vi "Fetch Single Measurement (Current Harmonics).vi"(0 "VISA resource name":refnum<visa-resource-name>, 7 "Harmonic Order (1)":u8=1, 9 "Phase Order (1)":u8=1, 11 "error in (no error)":errorcluster) -> (3 "Total Current Harmonic Distortion":dbl, 4 "VISA resource name out":refnum<visa-resource-name>, 6 "Current Crestfactor":dbl, 8 "Nth Current Harmonic Amplitude":dbl, 10 "Nth Current Harmonic Phase":dbl, 15 "error out":errorcluster)   [LabVIEW 2020, in "Agilent 681x Series.lvlib"]
doc: "Fetches and returns the selected order harmonic amplitude and phase measurements, the crestfactor of the waveform and the total harmonic distortion.\n\n<B>Note:</B>\n\nUse this VI only with other low-level VIs. The high-level VIs automatically incorporate this functionality. This VI does not check the instrument status. If you want to check the instrument status, call the Error Query VI at the conclusion of the sequence."
uses:
  <instrlib>/Agilent 681x Series/Agilent 681x Series.lvlib
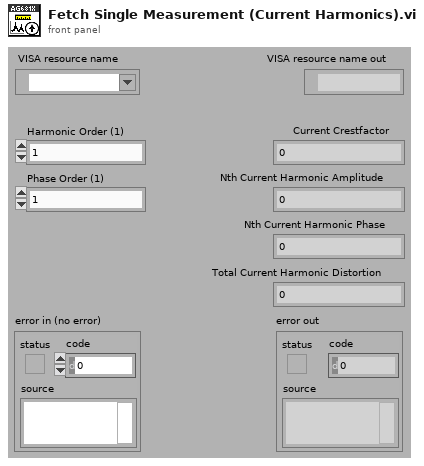
[diagram p1: front panel]
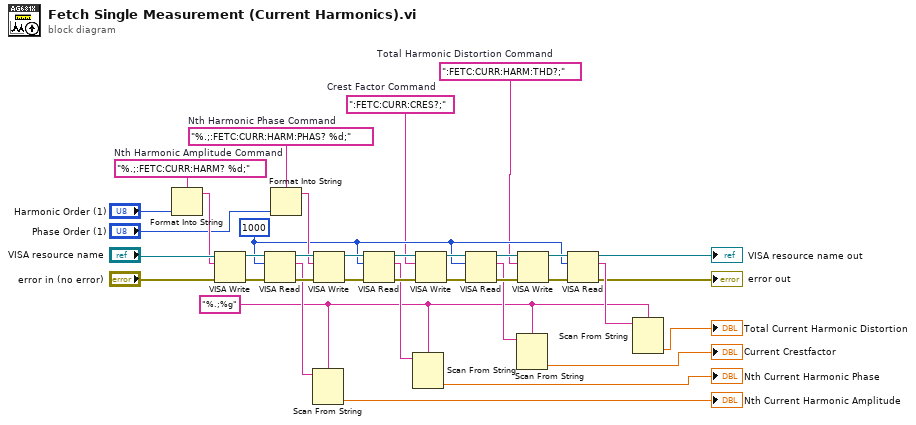
[diagram p0: block diagram]
diagram:
  w4 = "%.;%g" ("format string")
  w13 = ":FETC:CURR:CRES?;"  # Crest Factor Command
  w19 = "%.;:FETC:CURR:HARM:PHAS? %d;"  # Nth Harmonic Phase Command
  w20 = "%.;:FETC:CURR:HARM? %d;"  # Nth Harmonic Amplitude Command
  w14 = u32 1000 ("byte count")
  w12 = ":FETC:CURR:HARM:THD?;"  # Total Harmonic Distortion Command
  n1 = Format Into String(format string=w20, "Harmonic Order (1)") -> (resulting string=w17:string)  [unwired: 2 in, 1 out]
  n2 = VISA Write(VISA resource name="VISA resource name", write buffer=w17, error in (no error)="error in (no error)") -> (VISA resource name out=w33:refnum<visa-resource-name>, error out=w34:errorcluster)  [unwired: 1 out]
  n3 = VISA Read(VISA resource name=w33, byte count=w14, error in (no error)=w34) -> (VISA resource name out=w29:refnum<visa-resource-name>, read buffer=w5:string, error out=w30:errorcluster)  [unwired: 1 out]
  n4 = Format Into String(format string=w19, "Phase Order (1)") -> (resulting string=w16:string)  [unwired: 2 in, 1 out]
  n5 = Scan From String(format string=w4, input string=w5) -> (output 1=→"Nth Current Harmonic Amplitude":dbl)  [unwired: 3 in, 3 out]
  n6 = VISA Write(VISA resource name=w29, write buffer=w16, error in (no error)=w30) -> (VISA resource name out=w32:refnum<visa-resource-name>, error out=w31:errorcluster)  [unwired: 1 out]
  n7 = VISA Read(VISA resource name=w32, byte count=w14, error in (no error)=w31) -> (VISA resource name out=w25:refnum<visa-resource-name>, read buffer=w7:string, error out=w26:errorcluster)  [unwired: 1 out]
  n8 = Scan From String(format string=w4, input string=w7) -> (output 1=→"Nth Current Harmonic Phase":dbl)  [unwired: 3 in, 3 out]
  n9 = VISA Write(VISA resource name=w25, write buffer=w13, error in (no error)=w26) -> (VISA resource name out=w27:refnum<visa-resource-name>, error out=w28:errorcluster)  [unwired: 1 out]
  n10 = VISA Read(VISA resource name=w27, byte count=w14, error in (no error)=w28) -> (VISA resource name out=w21:refnum<visa-resource-name>, read buffer=w9:string, error out=w22:errorcluster)  [unwired: 1 out]
  n11 = Scan From String(format string=w4, input string=w9) -> (output 1=→"Current Crestfactor":dbl)  [unwired: 3 in, 3 out]
  n12 = VISA Write(VISA resource name=w21, write buffer=w12, error in (no error)=w22) -> (VISA resource name out=w24:refnum<visa-resource-name>, error out=w23:errorcluster)  [unwired: 1 out]
  n13 = VISA Read(VISA resource name=w24, byte count=w14, error in (no error)=w23) -> (VISA resource name out=→"VISA resource name out":refnum<visa-resource-name>, read buffer=w11:string, error out=→"error out":errorcluster)  [unwired: 1 out]
  n14 = Scan From String(format string=w4, input string=w11) -> (output 1=→"Total Current Harmonic Distortion":dbl)  [unwired: 3 in, 3 out]
